vi "报警信息通用.vi"(8 "error in (no error)":errorcluster, 10 "簇":T1, 11 "设备":string="环境动力") -> (0 "error out":errorcluster)   [LabVIEW 2016, in "环境动力监测库.lvlib"]
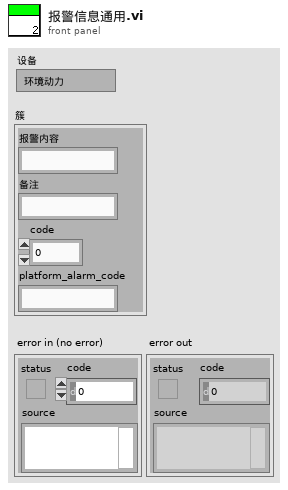
[diagram p1: front panel]
types:
  T1 = cluster{"报警内容":string, "备注":string, "code":i32, "platform_alarm_code":string}
  T2 = typedef "报警信息字段定义.ctl" = cluster{"时间":timestamp, "参数":string, "报警信息":string, "备注":string, "code":u64, "platform_alarm_code":string}
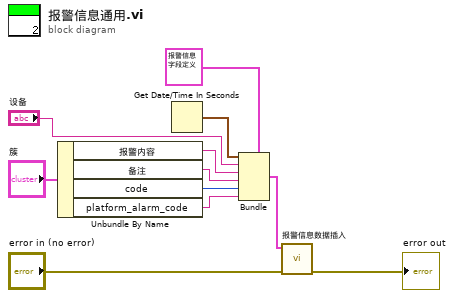
[diagram p0: block diagram]
diagram:
  n1 = Unbundle By Name("簇") -> ("报警内容"=w5:string, "备注"=w4:string, "code"=w2:i32, "platform_alarm_code"=w1:string)
  n2 = Get Date/Time In Seconds() -> (seconds since 1Jan1904=w11:timestamp)
  n3 = Bundle(cluster=T2 {"时间"=timestamp(0 s since 1904-01-01), "参数"="水样测试", "报警信息"="N", "备注"="", "code"=0, "platform_alarm_code"=""} ("data"), "时间"=w11, "参数"="设备", "报警信息"=w5, "备注"=w4, "code"=w2, "platform_alarm_code"=w1) -> (w9:T2)
  n4 = call "报警信息数据插入.vi"("data"=w9, "错误输入（无错误）"="error in (no error)") -> ("错误输出"=→"error out":errorcluster)  [unwired: 8 in]
